vi "Compute Maximum Desktop Bounds.vi"(8 "error in (no error)":errorcluster) -> (0 "error out":errorcluster, 1 "Max Panel Bounds":T3[](array[typedef]), 2 "Max Window Bounds":T3[](array[typedef]), 3 "All Monitor Positions":T2(array[cluster]))   [LabVIEW 2021, in "Panel Movement Center Maximize.lvlib"]
doc: "This VI will figure out the maximum bounds for that VI on all monitors. This computes how much space would be available if the VI were fully maximized, taking into account any platform limits such as a taskbar. Works on all operating systems. Returned will be an array of <b>All Monitor Positions</b>, all <b>Max Window Bounds</b> and all <b>Max Panel Bounds</b>. The first element in these arrays corresponds to the primary monitor.\n\nThis function perform a <b>Full Refresh</b> the first time it is called, and every subsequent call will return the last read values for the monitors and bounds. This decision was made because monitor positions, and resolutions aren't often changed after an application has started running. If this does occur, call this VI with the <b>Full Refresh</b> and the values will be recalculated.\n\nThis function runs in the UI thread.\n\n-----\nHooovahh\n(Brian Hoover)"
uses:
  <vilib>/Utility/miscctls.llb/LVRectTypeDef.ctl
  <vilib>/Utility/miscctls.llb/LVPositionTypeDef.ctl
  Panel Movement Center Maximize.lvlib
panel:
  in  "Position":T1
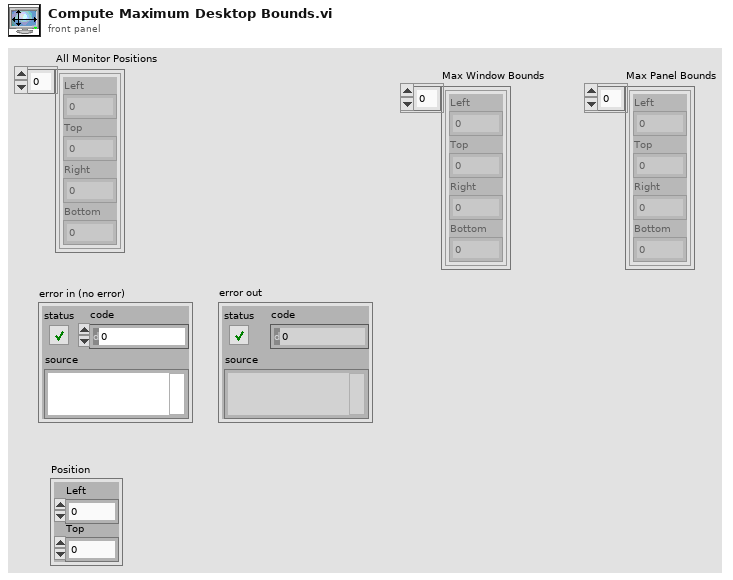
[diagram p1: front panel]
types:
  T1 = typedef "LVPositionTypeDef.ctl" = cluster{"Left":i32, "Top":i32}
  T2 = cluster{"Left":i16, "Top":i16, "Right":i16, "Bottom":i16}[]
  T3 = typedef "LVRectTypeDef.ctl" = cluster{"Left":i16, "Top":i16, "Right":i16, "Bottom":i16}
  T4 = enum32{"Invalid", "Standard", "Closed", "Hidden", "Minimized", "Maximized"}
  T5 = typedef "LVAllMonitorsDisplayTypeDef.ctl" = cluster{"Bounds":cluster{"Left":i16, "Top":i16, "Right":i16, "Bottom":i16}, "Depth":i16}[]
  T6 = cluster{"Left":i16, "Top":i16, "Right":i16, "Bottom":i16}
  T7 = cluster{"Left":bool, "Top":bool, "Right":bool, "Bottom":bool}
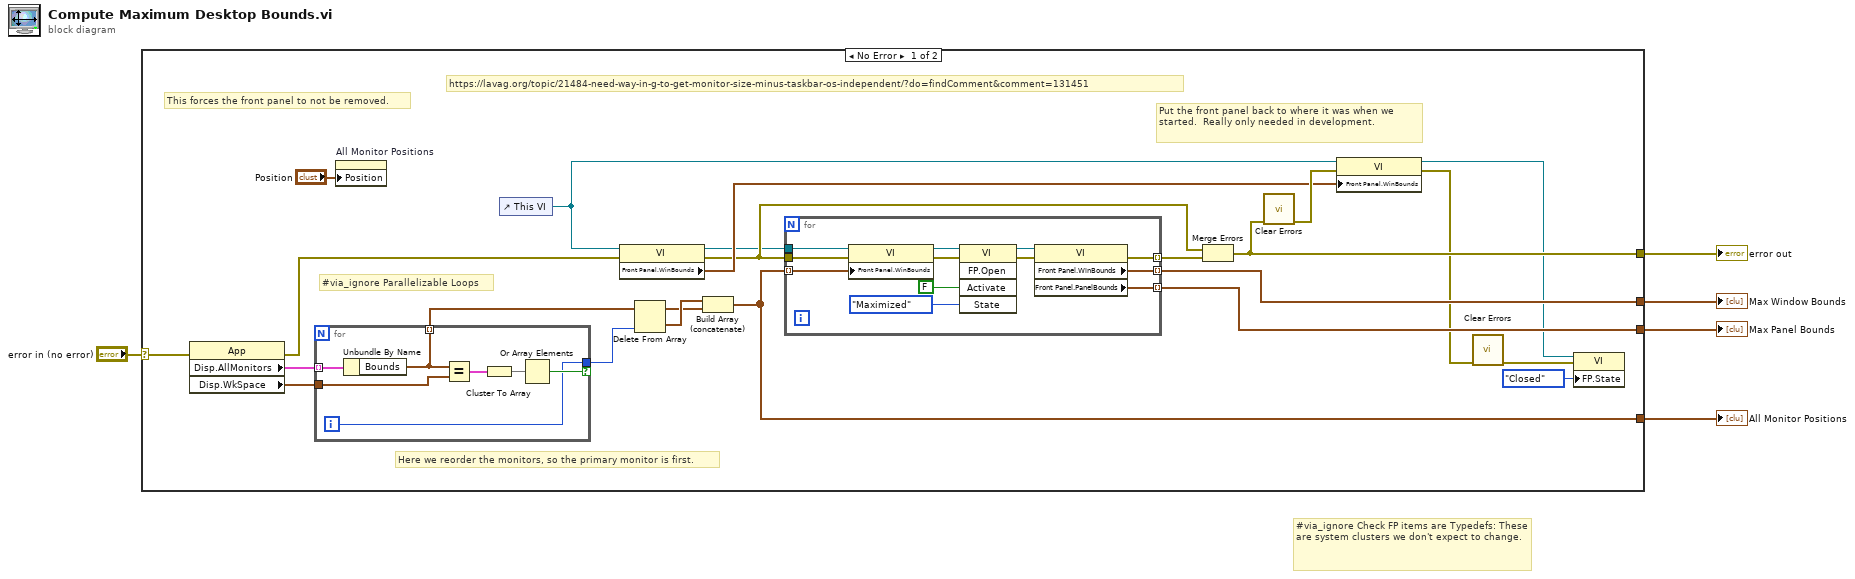
[diagram p0: block diagram]
diagram:
  # "#via_ignore Check FP items are Typedefs: These are system clusters we don't expect to change."
  n1 = case shown="No Error" "error in (no error)" {
    selector: "error in (no error)" -> [w28 w48]
    tunnel: [w27 w48] -> w4
    tunnel: [w26 _] -> w3
    tunnel: [w25 _] -> w2
    tunnel: [w24 _] -> w1
    frame No Error {
      # "This forces the front panel to not be removed."
      # "#via_ignore Parallelizable Loops"
      # "Here we reorder the monitors, so the primary monitor is first."
      # "Put the front panel back to where it was when we started.  Really only needed in development."
      # "https://lavag.org/topic/21484-need-way-in-g-to-get-monitor-size-minus-taskbar-os-independent/?do=findComment&comment=131451"
      n2 = property class="App"(error in=w28) -> (error out=w20:errorcluster, "Disp.AllMonitors"=w22:T5, "Disp.WkSpace"=w21:T3)  [unwired: 1 in, 1 out]
      n3 = for {
        tunnel: w22 -> [w47] mode=indexing
        tunnel: w21 -> [w46]
        tunnel: [w41] -> w14 if=w42
        tunnel: [w43] -> w17 mode=indexing
        i -> [w41]
        n4 = Unbundle By Name(w47) -> ("Bounds"=w43:T6)
        n5 = Equal?(x=w43, y=w46) -> (x = y?=w45:T7)
        n6 = Cluster To Array(cluster=w45) -> (array=w44:bool[])
        n7 = Or Array Elements(Boolean array=w44) -> (logical OR=w42:bool)
      }
      n8 = property on="All Monitor Positions" class="Arr (strict)"("Position"="Position") -> ()  [unwired: 2 in, 2 out]
      n9 = control-ref of="This VI"() -> (w11:refnum<vi>)
      n10 = property class="VI"(reference=w11, error in=w20) -> (reference out=w12:refnum<vi>, error out=w13:errorcluster, "Front Panel.WinBounds"=w18:T3)
      n11 = Delete From Array(array=w17, index=w14) -> (deleted portion=w16:T6, array with subset deleted=w15:T2)  [unwired: 1 in]
      n12 = Build Array (concatenate)(w16, w15) -> (w24:T2)
      n13 = for {
        tunnel: w24 -> [w40] mode=indexing
        tunnel: w13 -> [w34]
        tunnel: [w33] -> w23 mode=indexing
        tunnel: [w31] -> w26 mode=indexing
        tunnel: [w30] -> w25 mode=indexing
        tunnel: w12 -> [w29]
        n14 = property class="VI"(reference=w29, error in=w34, "Front Panel.WinBounds"=w40) -> (reference out=w35:refnum<vi>, error out=w36:errorcluster)
        n15 = invoke class="VI" method="FP.Open"(reference=w35, error in=w36, "Activate"=FALSE ("Activate?"), "State"=T4."Maximized") -> (reference out=w32:refnum<vi>, error out=w39:errorcluster)  [unwired: 1 in, 3 out]
        n16 = property class="VI"(reference=w32, error in=w39) -> (error out=w33:errorcluster, "Front Panel.WinBounds"=w31:T3, "Front Panel.PanelBounds"=w30:T3)  [unwired: 1 out]
      }
      n17 = Merge Errors(w13, w23) -> (w27:errorcluster)
      n18 = call <vilib>:"Clear Errors.vi"("error in (no error)"=w27) -> ("error out"=w19:errorcluster)  [unwired: 5 in, 1 out]
      n19 = property class="VI"(reference=w11, error in=w19, "Front Panel.WinBounds"=w18) -> (reference out=w10:refnum<vi>, error out=w8:errorcluster)
      n20 = call <vilib>:"Clear Errors.vi"("error in (no error)"=w8) -> ("error out"=w7:errorcluster)  [unwired: 5 in, 1 out]
      n21 = property class="VI"(reference=w10, error in=w7, "FP.State"=T4."Closed" ("Front Panel Window:State")) -> ()  [unwired: 2 out]
    }
    frame Error {
      # "#via_ignore CheckTunnelsUseDefaultValue"
      # "#via_ignore CheckTunnelsUseDefaultValue"
      # "#via_ignore CheckTunnelsUseDefaultValue"
    }
  }
  "error out" <- w4
  "Max Window Bounds" <- w3
  "Max Panel Bounds" <- w2
  "All Monitor Positions" <- w1
